vi "V7310.Variables.Get.vi"(6 "timeout ms (5000)":i32=5000, 8 "error in":errorcluster, 11 "Connection in":refnum<k5>) -> (0 "error out":errorcluster, 2 "Variables":string[](array[string]), 3 "Connection out":refnum<k5>)   [LabVIEW 2016]
uses:
  LowLevel/V7310.Commands.ctl
panel:
  out "Data out":string
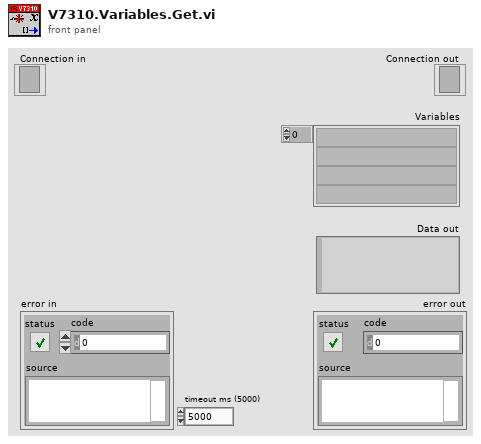
[diagram p1: front panel]
types:
  T1 = typedef "V7310.Commands.ctl" = enum16{"Start", "Stop", "GetStatus", "GetVarNames", "GetJobNames", "SetJob", "GetJob", "SetVars", "GetVars", "SetLayoutPosition", "SetRotation", "GetMessageID", "GetMessages", "ConfirmMessages", "DeleteMessages", "SetRTC", "GetRTC", "SetVarPosition", "SetIntensity", "GetIntensity", "SetStartTriggerDelay", "GetStartTriggerDelay", "SetStopTriggerDelay", "GetStopTriggerDelay", "SetConsecutiveTriggerDelay", "GetConsecutiveTriggerDelay", "SetMarkSpeed", "GetMarkSpeed"}
  T2 = typedef "V7310.ErrorLevels.ctl" = enum16{"OK", "Warning", "Error"}
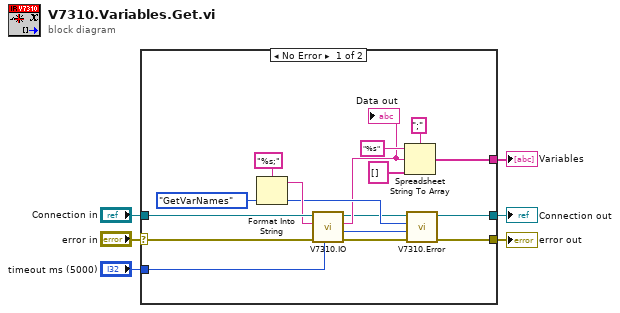
[diagram p0: block diagram]
diagram:
  n1 = case shown="No Error" "error in" {
    selector: "error in" -> [w20 w22]
    tunnel: "Connection in" -> [w21 w23]
    tunnel: [w10 w23] -> w5
    tunnel: "timeout ms (5000)" -> [w8 _]
    tunnel: [w9 w22] -> w2
    tunnel: [w7 _] -> w1
    frame No Error {
      w17 = V7310.Commands."GetVarNames" ("Cmd")
      n2 = Format Into String(format string="%s;", w17) -> (resulting string=w18:string)  [unwired: 2 in, 1 out]
      n3 = call "V7310.IO.vi"("timeout ms (5000)"=w8, "error in"=w20, "Data in"=w18, "Connection in"=w21) -> ("error out"=w15:errorcluster, "Error Level"=w16:T2, "Data out"=w11:string, "Connection out"=w10:refnum<k5>)  [unwired: 4 in]
      "Data out" <- w11
      n4 = Spreadsheet String To Array(delimiter (Tab)=";", format string="%s", spreadsheet string=w11, array type (2D Dbl)=string[] [] ("StrArray")) -> (array=w7:string[])
      n5 = call "V7310.Error.vi"("error in"=w15, "Error Level"=w16, "Cmd"=w17) -> ("error out"=w9:errorcluster)  [unwired: 8 in]
    }
    frame Error {
    }
  }
  "Connection out" <- w5
  "error out" <- w2
  "Variables" <- w1
